vi "Execute Transient.vi"() -> ()   [LabVIEW 2013]
uses:
  Instance           1 25Saved   Execute Transient .vi
panel:
  in  "Mode":bool=TRUE
  in  "Trans \nTime":dbl=1.0
  in  "Trans \nValue":dbl
  in  "Execute\nTransient":bool
  out "Total\nTime\nElapsed\n(sec)":u64=47
  in  "Log To File":bool
  in  "Cycles":bool caption="Single / Stop"
  out "Cycle\nTime\nElapsed\n(sec)":u64=7
  in  "Time/\nCycle \n(sec)":dbl=10.0
  out "Current vs Time":cluster{dbl[], dbl[]}(graph)
  out "Voltage vs Time":cluster{dbl[], dbl[]}(graph)
  in  "?":i32
  in  "VISA resource name":refnum<visa-resource-name>="GPIB0::6::INSTR"
  in  "Output":bool
  in  "?":i32
  out "error out":errorcluster
  in  "error in (no error)":errorcluster
  # "Continuous"
  # "Voltage"
  # "Current"
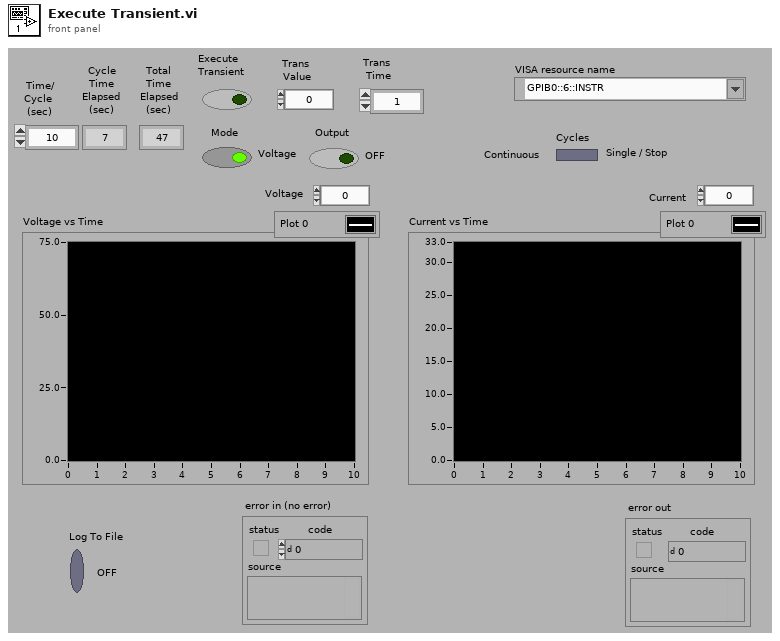
[diagram p1: front panel]
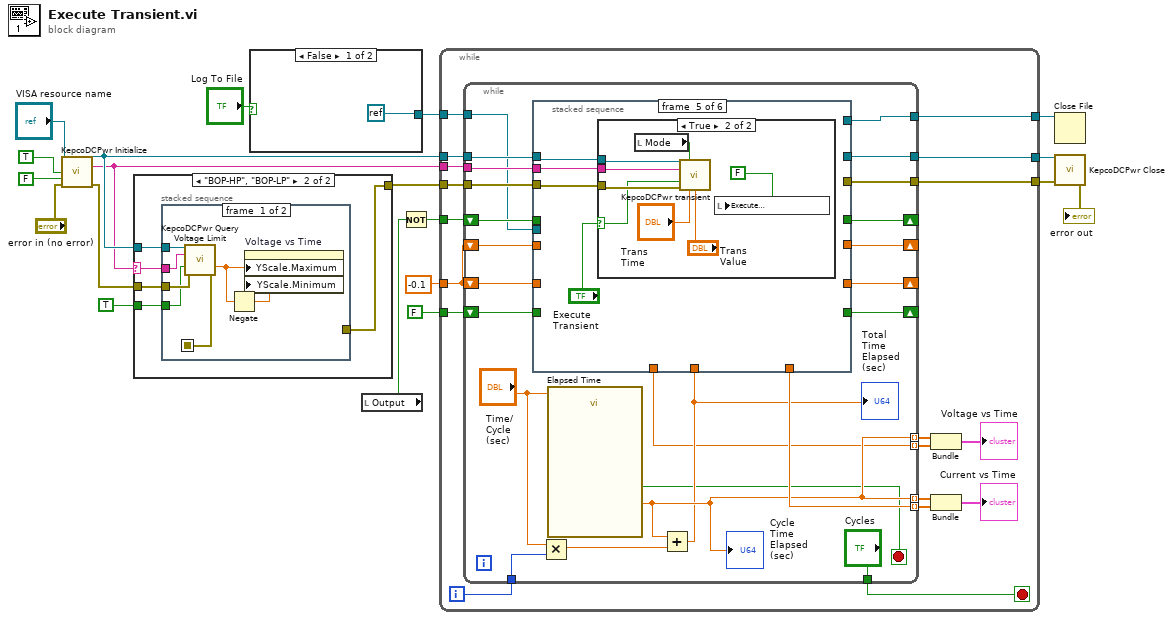
[diagram p0: block diagram]
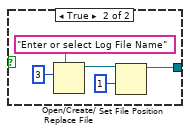
[diagram p2: hidden frame]
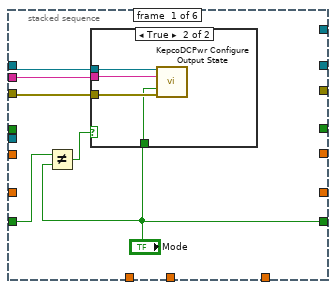
[diagram p3: hidden frame]
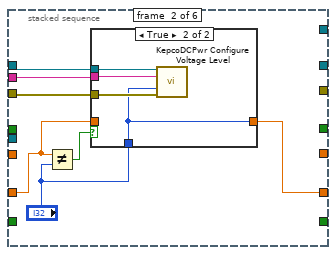
[diagram p5: hidden frame]
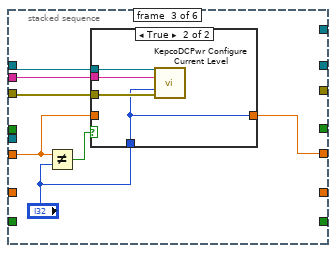
[diagram p7: hidden frame]
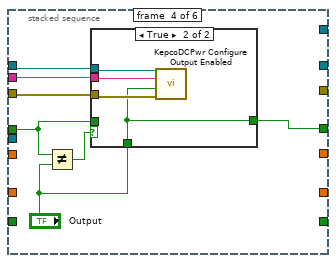
[diagram p9: hidden frame]
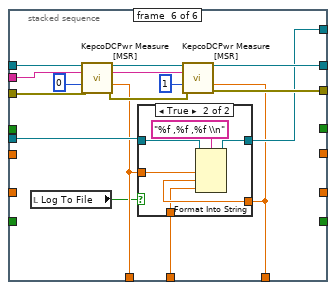
[diagram p12: hidden frame]
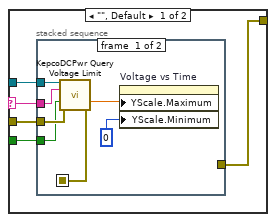
[diagram p14: hidden frame]
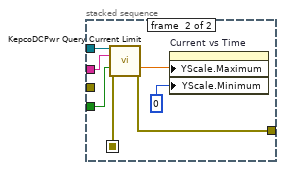
[diagram p15: hidden frame]
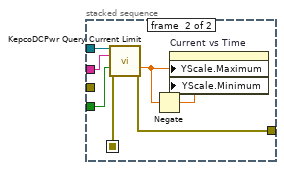
[diagram p16: hidden frame]
diagram:
  n1 = call "KepcoDCPwr Initialize.vi"("VISA Resource Name"="VISA resource name", "id query (True)"=TRUE, "reset device (True)"=FALSE ("id query (True)"), "error in (no error)"="error in (no error)") -> ("VISA Session Out"=w9:refnum<visa-resource-name>, "Model Out"=w8:string, "error out"=w7:errorcluster)  [unwired: 8 in, 1 out]
  n2 = case shown="\"BOP-HP\", \"BOP-LP\"" w8 {
    selector: w8 -> [w22 w41]
    tunnel: w9 -> [w24 w43]
    tunnel: w7 -> [w23 w42]
    tunnel: [w21 w40] -> w6
    tunnel: TRUE ("id query (True)") -> [w20 w39]
    frame "", Default {
      n3 = stacked-sequence {
        seq-local: [w26 _] -> [_ w34]
        tunnel: w24 -> [w31 w38]
        tunnel: w23 -> [w30 _]
        tunnel: w22 -> [w27 w35]
        tunnel: [_ w33] -> w21
        tunnel: w20 -> [w25 w32]
        frame #0 {
          n4 = call "KepcoDCPwr Query Voltage Limit.vi"("VISA Session"=w31, "Model In"=w27, "Max Level (T),MIN LEVEL(F)"=w25, "error in (no error)"=w30) -> ("voltage level"=w29:dbl, "error out"=w26:errorcluster)  [unwired: 7 in, 3 out]
          n5 = property on="Voltage vs Time" class="XYGraph (strict)"("YScale.Maximum"=w29, "YScale.Minimum"=0) -> ()  [unwired: 2 in, 2 out]
        }
        frame #1 {
          n6 = call "KepcoDCPwr Query Current Limit.vi"("VISA Session"=w38, "Model In"=w35, "Level"=w32, "error in (no error)"=w34) -> ("current limit"=w37:dbl, "error out"=w33:errorcluster)  [unwired: 7 in, 3 out]
          n7 = property on="Current vs Time" class="XYGraph (strict)"("YScale.Maximum"=w37, "YScale.Minimum"=0) -> ()  [unwired: 2 in, 2 out]
        }
      }
    }
    frame "BOP-HP", "BOP-LP" {
      n8 = stacked-sequence {
        seq-local: [w47 _] -> [_ w55]
        tunnel: w43 -> [w50 w57]
        tunnel: w42 -> [w49 _]
        tunnel: w41 -> [w48 w56]
        tunnel: [_ w54] -> w40
        tunnel: w39 -> [w46 w53]
        frame #0 {
          n9 = call "KepcoDCPwr Query Voltage Limit.vi"("VISA Session"=w50, "Model In"=w48, "Max Level (T),MIN LEVEL(F)"=w46, "error in (no error)"=w49) -> ("voltage level"=w44:dbl, "error out"=w47:errorcluster)  [unwired: 7 in, 3 out]
          n10 = Negate(x=w44) -> (-x=w45:dbl)
          n11 = property on="Voltage vs Time" class="XYGraph (strict)"("YScale.Maximum"=w44, "YScale.Minimum"=w45) -> ()  [unwired: 2 in, 2 out]
        }
        frame #1 {
          n12 = call "KepcoDCPwr Query Current Limit.vi"("VISA Session"=w57, "Model In"=w56, "Level"=w53, "error in (no error)"=w55) -> ("current limit"=w52:dbl, "error out"=w54:errorcluster)  [unwired: 7 in, 3 out]
          n13 = Negate(x=w52) -> (-x=w51:dbl)
          n14 = property on="Current vs Time" class="XYGraph (strict)"("YScale.Maximum"=w52, "YScale.Minimum"=w51) -> ()  [unwired: 2 in, 2 out]
        }
      }
    }
  }
  n15 = case shown="False" "Log To File" {
    tunnel: [refnum<k0> refnum w60] -> w4
    frame False {
    }
    frame True {
      n16 = Open/Create/Replace File(prompt="Enter or select Log File Name", operation (0:open)=3) -> (refnum out=w62:refnum<file>)  [unwired: 4 in, 2 out]
      n17 = Set File Position(refnum=w62, from (0:start)=1) -> (refnum out=w60:refnum<file>)  [unwired: 2 in, 1 out]
    }
  }
  n18 = local read "Output"() -> (w10:bool)
  n19 = Not(x=w10) -> (.not. x?=w11:bool)
  n20 = while {
    tunnel: [w81] -> w18
    tunnel: [w80] -> w17
    tunnel: -0.1 -> [w79]
    tunnel: w11 -> [w78]
    tunnel: w9 -> [w71]
    tunnel: w8 -> [w70]
    tunnel: w6 -> [w69]
    tunnel: w4 -> [w68]
    tunnel: [w67] -> w3
    tunnel: FALSE -> [w64]
    i -> [w66]
    stop <- w65 stop-if-true
    n21 = while {
      tunnel: w70 -> [w102]
      tunnel: w71 -> [w103]
      tunnel: w69 -> [w101]
      shift-right: [w105] -> _
      shift-left: w79 -> [w104]
      shift-right: [w100] -> _
      shift-left: w79 -> [w99]
      shift-right: [w97] -> _
      shift-left: w78 -> [w98]
      tunnel: [w96] -> w81
      tunnel: [w95] -> w80
      tunnel: [w84] -> w76 mode=indexing
      tunnel: [w91] -> w75 mode=indexing
      tunnel: [w94] -> w73 mode=indexing
      tunnel: [w91] -> w72 mode=indexing
      tunnel: w68 -> [w93]
      tunnel: [w92] -> w67
      tunnel: w66 -> [w90]
      tunnel: ["Cycles"] -> w65
      shift-right: [w83] -> _
      shift-left: w64 -> [w82]
      stop <- w87 stop-if-true
      n22 = Multiply(x="Time/\nCycle \n(sec)", y=w90) -> (x*y=w89:dbl)
      n23 = call "Elapsed Time"("Time Target (s)"="Time/\nCycle \n(sec)") -> ("Elapsed Time (s)"=w91:dbl, "Time has Elapsed"=w87:bool)  [unwired: 11 in, 6 out]
      "Cycle\nTime\nElapsed\n(sec)" <- w91
      n24 = Add(x=w91, y=w89) -> (x+y=w88:dbl)
      "Total\nTime\nElapsed\n(sec)" <- w88
      n25 = stacked-sequence {
        tunnel: [_ w118 _ _ _ _] -> w105
        tunnel: w104 -> [_ w117 _ _ _ _]
        tunnel: w103 -> [w111 w122 w133 w145 w155 w179]
        tunnel: w102 -> [w110 w121 w132 w144 w154 w178]
        tunnel: w101 -> [w109 w120 w131 w143 w153 w177]
        tunnel: [_ _ w129 _ _ _] -> w100
        tunnel: w99 -> [_ _ w128 _ _ _]
        tunnel: w98 -> [_ _ _ w140 _ _]
        tunnel: [_ _ _ w141 _ _] -> w97
        tunnel: [_ _ _ _ _ w171] -> w96
        tunnel: [_ _ _ _ _ w170] -> w95
        tunnel: [_ _ _ _ _ w167] -> w84
        tunnel: [_ _ _ _ _ w166] -> w94
        tunnel: w93 -> [_ _ _ _ _ w169]
        tunnel: [_ _ _ _ _ w168] -> w92
        tunnel: w88 -> [_ _ _ _ _ w165]
        tunnel: ["Mode" _ _ _ _ _] -> w83
        tunnel: w82 -> [w107 _ _ _ _ _]
        frame #0 {
          n26 = Not Equal?(x=w107, y="Mode") -> (x != y?=w108:bool)
          n27 = case shown="True" w108 {
            tunnel: w111 -> [_ w115]
            tunnel: w110 -> [_ w114]
            tunnel: w109 -> [_ w113]
            tunnel: "Mode" -> [_ w112]
            frame False {
            }
            frame True {
              n28 = call "KepcoDCPwr Configure Output State.vi"("VISA Session"=w115, "Model In"=w114, "Power Supply Mode"=w112, "error in (no error)"=w113) -> ()  [unwired: 8 in, 4 out]
            }
          }
        }
        frame #1 {
          n29 = Not Equal?(x=w117, y="?") -> (x != y?=w116:bool)
          n30 = case shown="True" w116 {
            tunnel: w122 -> [_ w127]
            tunnel: w121 -> [_ w126]
            tunnel: w120 -> [_ w125]
            tunnel: "?" -> [_ w124]
            tunnel: [w123 w124] -> w118
            tunnel: w117 -> [w123 _]
            frame False {
            }
            frame True {
              n31 = call "KepcoDCPwr Configure Voltage Level.vi"("VISA Session"=w127, "Model In"=w126, "level (0.0 volts)"=w124, "error in (no error)"=w125) -> ()  [unwired: 8 in, 4 out]
            }
          }
        }
        frame #2 {
          n32 = Not Equal?(x=w128, y="?") -> (x != y?=w134:bool)
          n33 = case shown="True" w134 {
            tunnel: w133 -> [_ w139]
            tunnel: w132 -> [_ w138]
            tunnel: w131 -> [_ w137]
            tunnel: "?" -> [_ w136]
            tunnel: [w135 w136] -> w129
            tunnel: w128 -> [w135 _]
            frame False {
            }
            frame True {
              n34 = call "KepcoDCPwr Configure Current Level.vi"("VISA Session"=w139, "Model In"=w138, "level (0.0 volts)"=w136, "error in (no error)"=w137) -> ()  [unwired: 8 in, 4 out]
            }
          }
        }
        frame #3 {
          n35 = Not Equal?(x=w140, y="Output") -> (x != y?=w146:bool)
          n36 = case shown="True" w146 {
            tunnel: w145 -> [_ w149]
            tunnel: w144 -> [_ w151]
            tunnel: w143 -> [_ w150]
            tunnel: "Output" -> [_ w148]
            tunnel: [w147 w148] -> w141
            tunnel: w140 -> [w147 _]
            frame False {
            }
            frame True {
              n37 = call "KepcoDCPwr Configure Output Enabled.vi"("VISA Session"=w149, "Model In"=w151, "Input enabled (True)"=w148, "error in (no error)"=w150) -> ()  [unwired: 9 in, 3 out]
            }
          }
        }
        frame #4 {
          n38 = case shown="True" "Execute\nTransient" {
            selector: "Execute\nTransient" -> [_ w160]
            tunnel: w155 -> [_ w161]
            tunnel: w154 -> [_ w163]
            tunnel: w153 -> [_ w162]
            frame False {
            }
            frame True {
              n39 = local read "Mode"() -> (w156:bool)
              n40 = call "KepcoDCPwr transient.vi"("VISA Session"=w161, "Mode"=w156, "Model In"=w163, "Trans Enabled"=w160, "error in (no error)"=w162, "Trans Time"="Trans \nTime", "Trans Value"="Trans \nValue") -> ()  [unwired: 5 in, 4 out]
              n41 = local write "Execute\nTransient"(FALSE) -> ()
            }
          }
        }
        frame #5 {
          n42 = local read "Log To File"() -> (w164:bool)
          n43 = call "KepcoDCPwr Measure [MSR].vi"("VISA Session"=w179, "Model In"=w178, "measurement type (voltage)"=0, "error in (no error)"=w177) -> ("VISA Session Out"=w175:refnum<visa-resource-name>, "Model Out"=w174:string, "measurement"=w167:dbl, "error out"=w172:errorcluster)  [unwired: 7 in, 1 out]
          n44 = call "KepcoDCPwr Measure [MSR].vi"("VISA Session"=w175, "Model In"=w174, "measurement type (voltage)"=1, "error in (no error)"=w172) -> ("VISA Session Out"=w171:refnum<visa-resource-name>, "measurement"=w166:dbl, "error out"=w170:errorcluster)  [unwired: 7 in, 2 out]
          n45 = case shown="True" w164 {
            tunnel: w169 -> [w180 w185]
            tunnel: [w180 w184] -> w168
            tunnel: w167 -> [_ w183]
            tunnel: w166 -> [_ w182]
            tunnel: w165 -> [_ w181]
            frame False {
            }
            frame True {
              n46 = Format Into String(format string="%f ,%f ,%f \\n", initial string=w185, w183, w182, w181) -> (resulting string=w184:refnum<file>)  [unwired: 1 in, 1 out]
            }
          }
        }
      }
    }
    n47 = Bundle(w75, w76) -> (→"Voltage vs Time":cluster{dbl[], dbl[]})  [unwired: 1 in]
    n48 = Bundle(w72, w73) -> (→"Current vs Time":cluster{dbl[], dbl[]})  [unwired: 1 in]
  }
  n49 = Close File(refnum=w3) -> ()  [unwired: 1 in, 2 out]
  n50 = call "KepcoDCPwr Close.vi"("VISA Session"=w18, "error in (no error)"=w17) -> ("error out"=→"error out":errorcluster)  [unwired: 13 in]
